vi "Read or Write Configurations.vi"(0 "Architecture":string, 5 "Maintainer":string, 7 "Email":string, 11 "error in (no error)":errorcluster, 13 "Operation":T1) -> (4 "Architecture Out":string, 6 "Maintainer Out":string, 8 "Email Out":string, 15 "error out":errorcluster)   [LabVIEW 2021, in "Packager Helpers.lvlib"]
uses:
  Packager Helpers.lvlib
  controls/Config File Operations.ctl
  <vilib>/Utility/config.llb/Read Key (String).vi
  <vilib>/Utility/config.llb/Write Key (String).vi
  <vilib>/Utility/config.llb/NI_LVConfig.lvlib
  Path Functions/Path Functions.lvlib
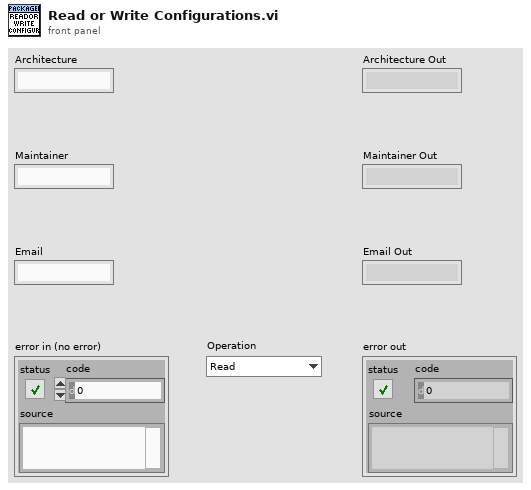
[diagram p1: front panel]
types:
  T1 = typedef "Packager Helpers.lvlib/Config File Operations.ctl" = enum16{"Read", "Write"}
  T2 = typedef "NI_LVConfig.lvlib/Config Data RefNum.ctl" = refnum<k1>
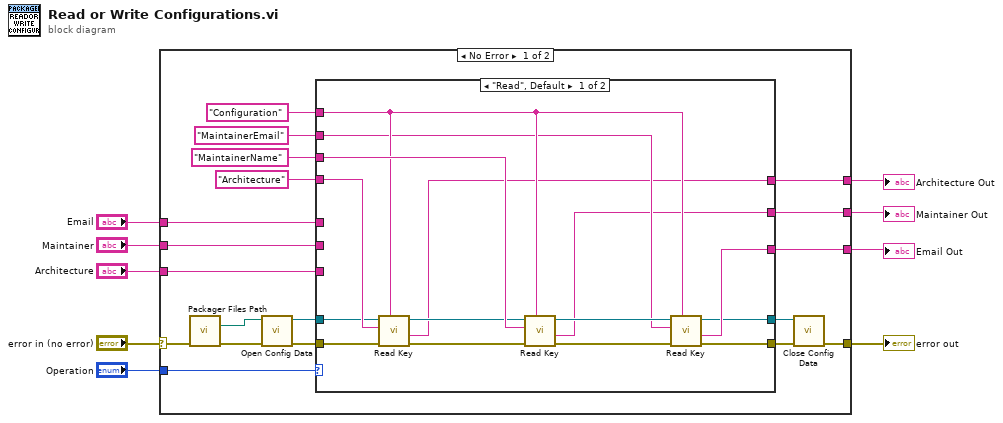
[diagram p0: block diagram]
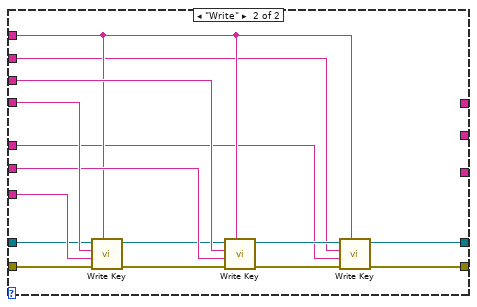
[diagram p2: hidden frame]
diagram:
  n1 = case shown="No Error" "error in (no error)" {
    selector: "error in (no error)" -> [w14 w59]
    tunnel: "Operation" -> [w16 _]
    tunnel: [w22 _] -> w8
    tunnel: [w21 _] -> w7
    tunnel: [w20 _] -> w6
    tunnel: "Architecture" -> [w19 _]
    tunnel: "Maintainer" -> [w18 _]
    tunnel: "Email" -> [w17 _]
    tunnel: [w10 w59] -> w2
    frame No Error {
      n2 = call "Packager Files Path.vi"("error in (no error)"=w14) -> ("Config File Path"=w28:path, "error out"=w13:errorcluster)  [unwired: 12 in, 1 out]
      n3 = call <vilib>:"Open Config Data.vi"("error in (no error)"=w13, "configuration file path"=w28) -> ("error out"=w11:errorcluster, "refnum"=w12:T2)  [unwired: 7 in, 1 out]
      n4 = case shown="\"Read\", Default" w16 {
        tunnel: w11 -> [w33 w47]
        tunnel: "Configuration" ("section") -> [w41 w55]
        tunnel: "Architecture" ("section") -> [w43 w58]
        tunnel: "MaintainerName" ("section") -> [w42 w57]
        tunnel: "MaintainerEmail" ("section") -> [w38 w52]
        tunnel: [w30 w44] -> w15
        tunnel: [w37 _] -> w20
        tunnel: [w36 _] -> w21
        tunnel: [w35 _] -> w22
        tunnel: [w34 w54] -> w23
        tunnel: w19 -> [_ w49]
        tunnel: w18 -> [_ w56]
        tunnel: w17 -> [_ w51]
        tunnel: w12 -> [w29 w48]
        frame "Read", Default {
          n5 = call-poly <vilib>:"Read Key.vi"("section"=w41, "error in (no error)"=w33, "key"=w43, "refnum"=w29) -> ("error out"=w32:errorcluster, "value"=w35:string, "refnum out"=w39:T2)  [unwired: 4 in, 1 out]
          n6 = call-poly <vilib>:"Read Key.vi"("section"=w41, "error in (no error)"=w32, "key"=w42, "refnum"=w39) -> ("error out"=w31:errorcluster, "value"=w36:string, "refnum out"=w40:T2)  [unwired: 4 in, 1 out]
          n7 = call-poly <vilib>:"Read Key.vi"("section"=w41, "error in (no error)"=w31, "key"=w38, "refnum"=w40) -> ("error out"=w30:errorcluster, "value"=w37:string, "refnum out"=w34:T2)  [unwired: 4 in, 1 out]
        }
        frame "Write" {
          n8 = call-poly <vilib>:"Write Key.vi"("section"=w55, "error in (no error)"=w47, "value"=w49, "key"=w58, "refnum"=w48) -> ("error out"=w46:errorcluster, "refnum out"=w50:T2)  [unwired: 4 in, 1 out]
          n9 = call-poly <vilib>:"Write Key.vi"("section"=w55, "error in (no error)"=w46, "value"=w56, "key"=w57, "refnum"=w50) -> ("error out"=w45:errorcluster, "refnum out"=w53:T2)  [unwired: 4 in, 1 out]
          n10 = call-poly <vilib>:"Write Key.vi"("section"=w55, "error in (no error)"=w45, "value"=w51, "key"=w52, "refnum"=w53) -> ("error out"=w44:errorcluster, "refnum out"=w54:T2)  [unwired: 4 in, 1 out]
        }
      }
      n11 = call <vilib>:"Close Config Data.vi"("error in (no error)"=w15, "refnum"=w23) -> ("error out"=w10:errorcluster)  [unwired: 8 in, 1 out]
    }
    frame Error {
    }
  }
  "error out" <- w2
  "Email Out" <- w6
  "Maintainer Out" <- w7
  "Architecture Out" <- w8
